vi "FTW-TransferClient-S3-Callback-Progress.vi"(4 "Initial Params":T1, 5 "Event Data":cluster{"sender":refnum<k24>, "e":refnum<k24>}, 6 "Control Ref":refnum<k24>, 7 "Event Common Data":T2) -> ()   [LabVIEW 2012, in "FTW-TransferClient-S3.lvclass"]
uses:
  FTW-TransferClient-S3.lvclass
  C:/Users/Jack/repo/ftw-master/Web/Transfer Client/S3/AWSSDK.dll
  AWSSDK.dll
  FTW-TransferClient-TransferProgress.ctl
  FTW-TransferClient.lvclass
panel:
  # "Inputs"
  # "Outputs"
  # "No Outputs - this VI\nis fire and forget"
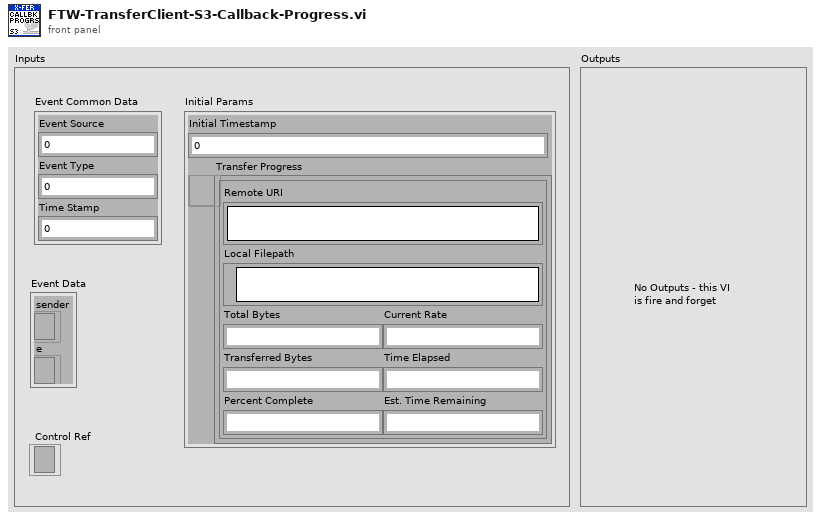
[diagram p1: front panel]
types:
  T1 = cluster{"Initial Timestamp":u32, "Transfer Progress":refnum<user-event>}
  T2 = cluster{"Event Source":i32, "Event Type":u32, "Time Stamp":u32}
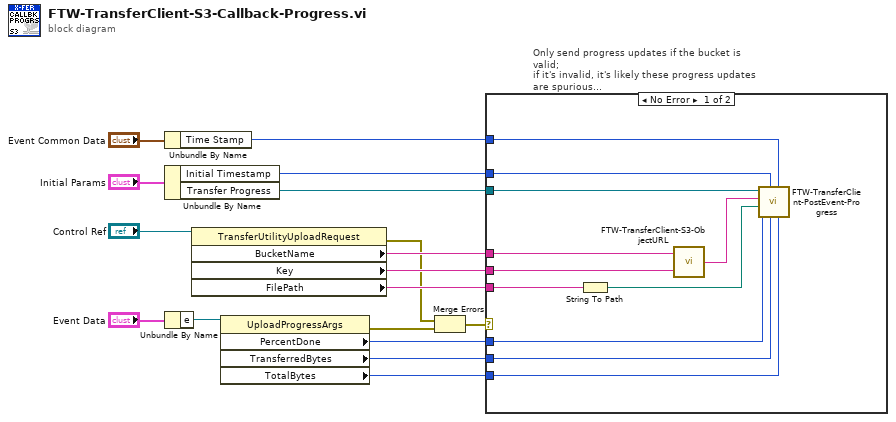
[diagram p0: block diagram]
diagram:
  n1 = Unbundle By Name("Event Common Data") -> ("Time Stamp"=w11:u32)
  n2 = Unbundle By Name("Initial Params") -> ("Initial Timestamp"=w12:u32, "Transfer Progress"=w10:refnum<user-event>)
  n3 = Unbundle By Name("Event Data") -> ("e"=w17:refnum<k24>)
  n4 = property class="TransferUtilityUploadRequest"(reference="Control Ref") -> (error out=w2:errorcluster, "BucketName"=w4:string, "Key"=w8:string, "FilePath"=w13:string)  [unwired: 1 in, 1 out]
  n5 = property class="UploadProgressArgs"(reference=w17) -> (error out=w1:errorcluster, "PercentDone"=w6:i32, "TransferredBytes"=w9:i64, "TotalBytes"=w5:i64)  [unwired: 1 in, 1 out]
  n6 = Merge Errors(w2, w1) -> (w3:errorcluster)
  n7 = case "Only send progress updates if the bucket is valid;\nif it's invalid, it's likely these progress updates are spurious\nattempts to contact the server" shown="No Error" w3 {
    tunnel: w13 -> [w28 _]
    tunnel: w12 -> [w27 _]
    tunnel: w11 -> [w26 _]
    tunnel: w10 -> [w25 _]
    tunnel: w9 -> [w24 _]
    tunnel: w8 -> [w23 _]
    tunnel: w6 -> [w22 _]
    tunnel: w5 -> [w21 _]
    tunnel: w4 -> [w20 _]
    frame No Error {
      n8 = String To Path(string=w28) -> (path=w19:path)
      n9 = call "FTW-TransferClient-S3-ObjectURL.vi"("Object Bucket"=w20, "Object Key"=w23) -> ("Object URL"=w18:string)  [unwired: 2 in]
      n10 = call "FTW-TransferClient-PostEvent-Progress.vi"("TotalBytes"=w21, "Timestamp"=w26, "TransferredBytes"=w24, "Initial Timestamp"=w27, "Percent Done"=w22, "Local Filepath"=w19, "Remote URI"=w18, "Transfer Progress Event"=w25) -> ()  [unwired: 4 in]
    }
    frame Error {
    }
  }
